vi "A170316-11_IO.vi"() -> ()   [LabVIEW 2020]
uses:
  TCP/S7Ref.vi
panel:
  in  "Q 3":T1
  in  "选项卡控件":enum32{"数字量输入", "数字量输出", "模拟量/伺服"}(tab)
  out "I 0":T2
  out "I 1":T3
  out "I 2":T3
  out "I 3":T3
  in  "Q 2":T1
  in  "Q 0":T4
  in  "Q 1":T1
  # "激光打标机"
  # "/"
  # "蜗杆伺服"
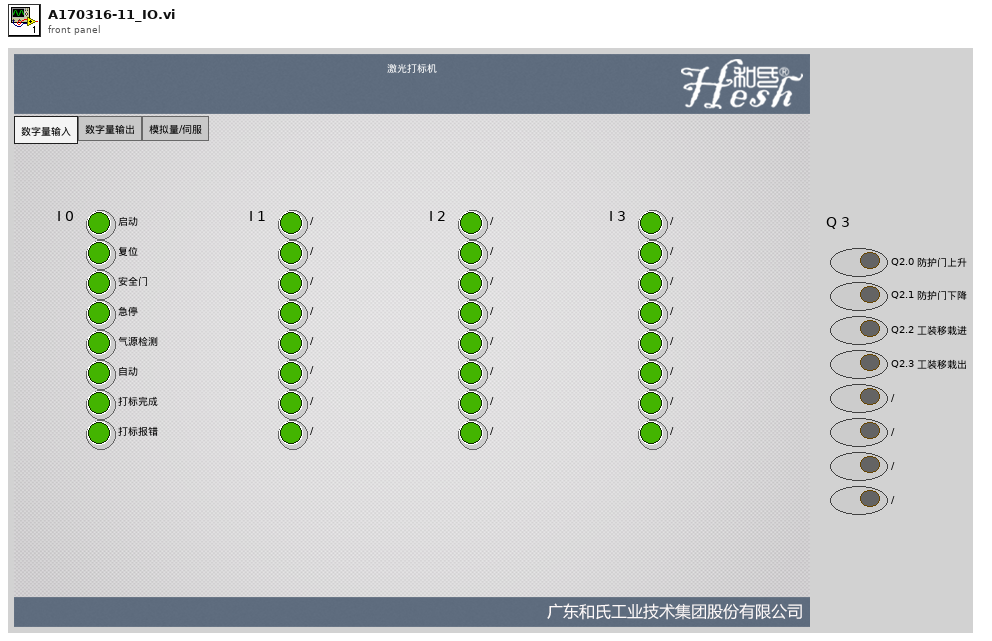
[diagram p1: front panel]
types:
  T1 = cluster{bool, bool, bool, bool, "/":bool, "/":bool, "/":bool, "/":bool}
  T2 = cluster{"启动":bool, "复位":bool, "安全门":bool, "急停":bool, "气源检测":bool, "自动":bool, "打标完成":bool, "打标报错":bool}
  T3 = cluster{"/":bool, "/":bool, "/":bool, "/":bool, "/":bool, "/":bool, "/":bool, "/":bool}
  T4 = cluster{"Q0.0启动打标":bool, "Q0.1":bool, bool, bool, "绿灯":bool, "/":bool, "/":bool, bool}
  T5 = cluster{bool, bool, bool, bool, bool, bool, bool, bool}
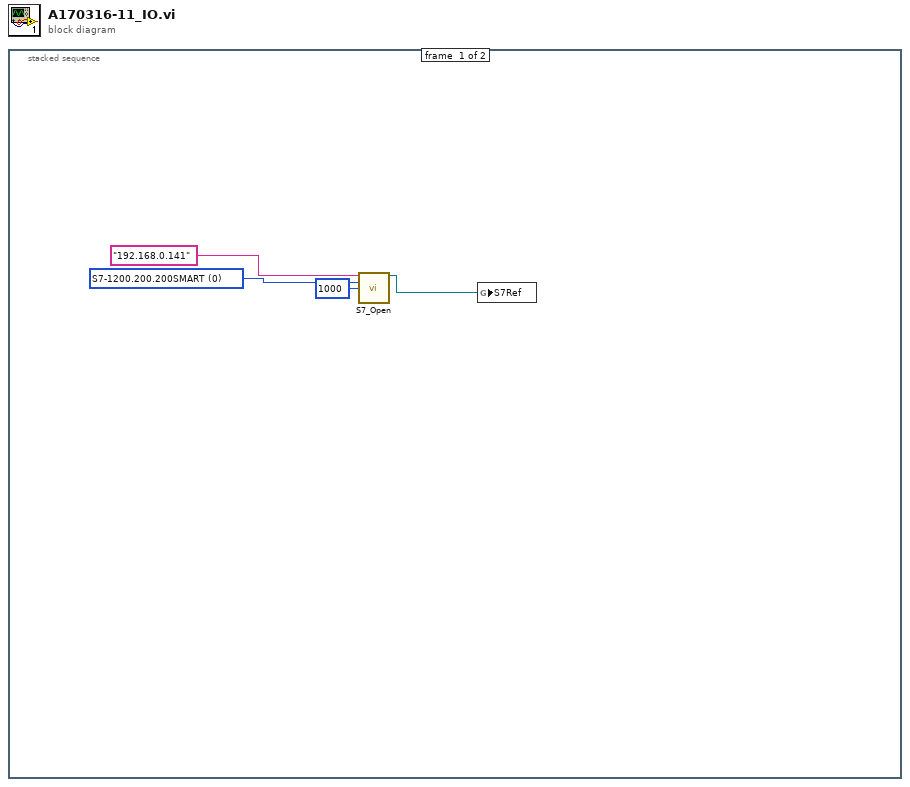
[diagram p0: block diagram]
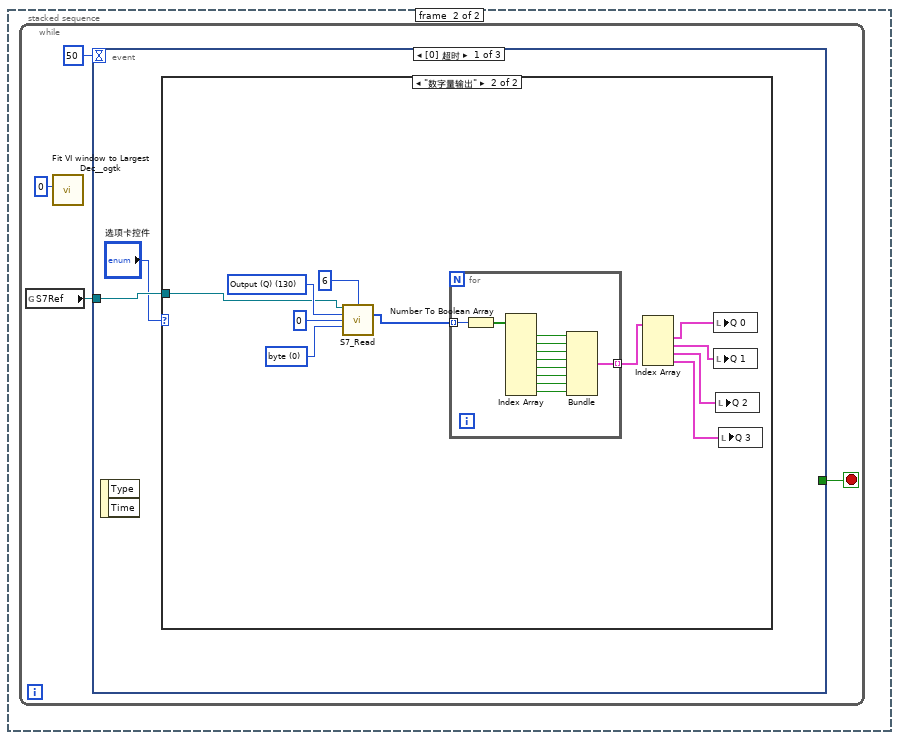
[diagram p2: hidden frame]
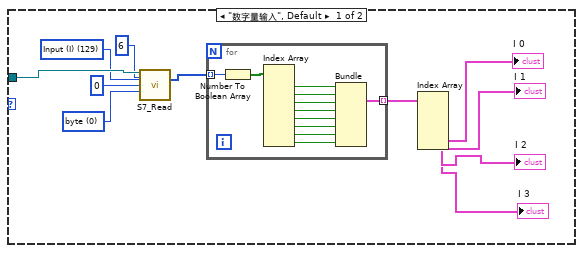
[diagram p3: hidden frame]
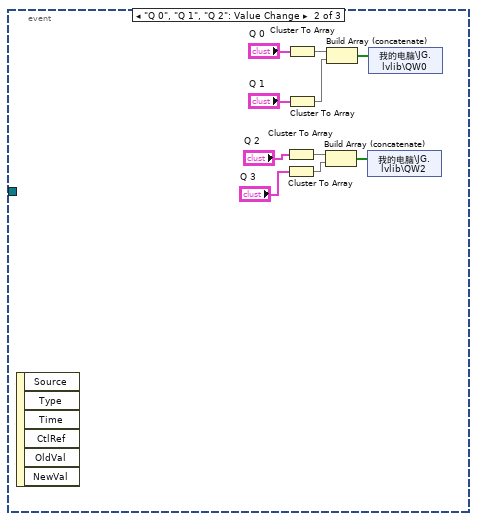
[diagram p4: hidden frame]
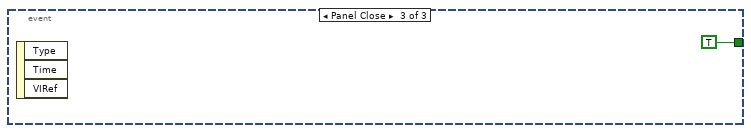
[diagram p5: hidden frame]
diagram:
  n1 = stacked-sequence {
    frame #0 {
      w2 = u8 0 items=["S7-1200.200.200SMART"=0, "S7-300"=2, "S7-400"=3] ("PLC 系列")
      n2 = call "S7_Open .vi"("IP 地址"="192.168.0.141", "PLC 系列"=w2, "超时（MS）"=1000) -> ("TCP"=w4:refnum<k5>)  [unwired: 9 in, 3 out]
      n3 = global write "S7Ref.vi" "S7Ref"(w4) -> ()
    }
    frame #1 {
      n4 = while {
        stop <- w8 stop-if-true
        n5 = global read "S7Ref.vi" "S7Ref"() -> (w5:refnum<k5>)
        n6 = call <userlib>:"Fit VI window to Largest Dec__ogtk.vi"("border spacing (2 px)"=0) -> ()  [unwired: 5 in, 2 out]
        n7 = event shown="[0] 超时" {
          selector: _ -> [_ _ _]
          dyn-events: _ -> [_ _ _]
          timeout: 50 -> [_ _ _]
          tunnel: [_ _ TRUE] -> w8
          tunnel: w5 -> [w10 _ _]
          event Timeout {
            n8 = event-data() -> ()  [unwired: 1 in, 2 out]
            n9 = case shown="\"数字量输出\"" "选项卡控件" {
              tunnel: w10 -> [w21 w39]
              frame "数字量输入", Default {
                w18 = u16 0 items=["byte", "word", "Dword"] ("数据类型")
                w20 = u8 129 items=["I/O (P)"=128, "Input (I)"=129, "Output (Q)"=130, "Bit Memory (M)"=131, "Data (DB)"=132, "Instance Data (DI)"=133, "Local Data (L)"=134, "Predecessor Local Data (VL)"=135] ("寄存器类型")
                n10 = call "S7_Read.vi"("TCP"=w21, "读取长度"=u16 6, "寄存器类型"=w20, "起始地址"=u32 0, "数据类型"=w18) -> ("数据"=w16:u32[])  [unwired: 7 in, 3 out]
                n11 = for {
                  tunnel: w16 -> [w32] mode=indexing
                  tunnel: [w26] -> w15 mode=indexing
                  n12 = Number To Boolean Array(number=w32) -> (Boolean array=w31:bool[])
                  n13 = Index Array(array=w31) -> (element #1=w30:bool, element #2=w29:bool, element #3=w28:bool, element #4=w27:bool, element #5=w25:bool, element #6=w24:bool, element #7=w23:bool, element #8=w22:bool)  [unwired: 8 in]
                  n14 = Bundle(w30, w29, w28, w27, w25, w24, w23, w22) -> (w26:T5)  [unwired: 1 in]
                }
                n15 = Index Array(array=w15) -> (element #1=→"I 0":T5, element #2=→"I 1":T5, element #4=→"I 2":T5, element #5=→"I 3":T5)  [unwired: 5 in, 1 out]
              }
              frame "数字量输出" {
                w40 = u16 0 items=["byte", "word", "Dword"] ("数据类型")
                w42 = u8 130 items=["I/O (P)"=128, "Input (I)"=129, "Output (Q)"=130, "Bit Memory (M)"=131, "Data (DB)"=132, "Instance Data (DI)"=133, "Local Data (L)"=134, "Predecessor Local Data (VL)"=135] ("寄存器类型")
                n16 = call "S7_Read.vi"("TCP"=w39, "读取长度"=u16 6, "寄存器类型"=w42, "起始地址"=u32 0, "数据类型"=w40) -> ("数据"=w38:u32[])  [unwired: 7 in, 3 out]
                n17 = for {
                  tunnel: w38 -> [w54] mode=indexing
                  tunnel: [w44] -> w37 mode=indexing
                  n18 = Number To Boolean Array(number=w54) -> (Boolean array=w53:bool[])
                  n19 = Index Array(array=w53) -> (element #1=w52:bool, element #2=w51:bool, element #3=w50:bool, element #4=w49:bool, element #5=w48:bool, element #6=w47:bool, element #7=w46:bool, element #8=w45:bool)  [unwired: 8 in]
                  n20 = Bundle(w52, w51, w50, w49, w48, w47, w46, w45) -> (w44:T5)  [unwired: 1 in]
                }
                n21 = Index Array(array=w37) -> (element #1=w36:T5, element #2=w35:T5, element #3=w34:T5, element #4=w33:T5)  [unwired: 4 in]
                n22 = local write "Q 0"(w36) -> ()
                n23 = local write "Q 1"(w35) -> ()
                n24 = local write "Q 2"(w34) -> ()
                n25 = local write "Q 3"(w33) -> ()
              }
            }
          }
          event "Q 0", "Q 1", "Q 2": Value Change {
            n26 = event-data() -> ()  [unwired: 1 in, 6 out]
            n27 = Cluster To Array(cluster="Q 2") -> (array=w59:bool[])
            n28 = Cluster To Array(cluster="Q 3") -> (array=w56:bool[])
            n29 = Cluster To Array(cluster="Q 0") -> (array=w62:bool[])
            n30 = Cluster To Array(cluster="Q 1") -> (array=w61:bool[])
            n31 = Build Array (concatenate)(w59, w56) -> (w58:bool[])
            n32 = Build Array (concatenate)(w62, w61) -> (w60:bool[])
            n33 = shared-variable "我的电脑\\JG.lvlib\\QW2"(w58) -> ()  [unwired: 1 in, 1 out]
            n34 = shared-variable "我的电脑\\JG.lvlib\\QW0"(w60) -> ()  [unwired: 1 in, 1 out]
          }
          event Panel Close {
            n35 = event-data() -> ()  [unwired: 1 in, 3 out]
          }
        }
      }
    }
  }
